vi "CloseConnection.vi"(8 "error in (no error)":errorcluster, 11 "MongoDB-Client in":refnum<class "MongoDB-Client.lvclass">) -> (0 "error out":errorcluster)   [LabVIEW 2016, in "MongoDB-Client.lvlib" / "MongoDB-Client.lvclass"]
uses:
  MongoDB-Client.lvclass
  D:/Users/blume/Desktop/LV/MongoDB-Driver/MLV DLLs/MongoLabVIEW.dll
  LV/MongoDB-Driver/MLV DLLs/MongoLabVIEW.dll
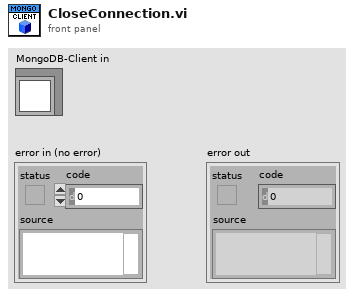
[diagram p1: front panel]
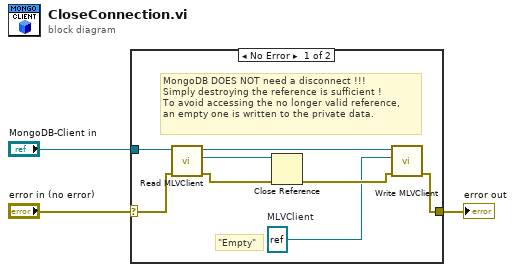
[diagram p0: block diagram]
diagram:
  n1 = case shown="No Error" "error in (no error)" {
    selector: "error in (no error)" -> [w10 w12]
    tunnel: [w6 w12] -> w2
    tunnel: "MongoDB-Client in" -> [w11 _]
    frame No Error {
      w4 = refnum<k24> refnum  # MLVClient
      # "\"Empty\""
      # "MongoDB DOES NOT need a disconnect !!!\nSimply destroying the reference is sufficient !\nTo avoid accessing the no longer valid reference,\nan empty one is written to the private data."
      n2 = call "Read MLVClient.vi"("error in (no error)"=w10, "MongoDB-Client in"=w11) -> ("error out"=w8:errorcluster, "MLVClient"=w9:refnum<k24>, "MongoDB-Client out"=w7:refnum<class "MongoDB-Client.lvclass">)  [unwired: 7 in]
      n3 = Close Reference(reference=w9, error in (no error)=w8) -> (error out=w5:errorcluster)
      n4 = call "Write MLVClient.vi"("error in (no error)"=w5, "MLVClient"=w4, "MongoDB-Client in"=w7) -> ("error out"=w6:errorcluster)  [unwired: 7 in, 1 out]
    }
    frame Error {
    }
  }
  "error out" <- w2
